vi "VarientToProperties.vi"(8 "error in (no error)":errorcluster, 11 "AcPwrPlugins.lvlib:NHRDCModel.lvclass":refnum<class "NHRDCPowerModel.lvclass">) -> (0 "error out":errorcluster, 1 "Measurements":T1, 2 "Device(s)Settings":T3 {"Modules"."Regulation Gain (1=100%)" min=0.0 max=1.0; "Modules"."OutputSettings"."Wait on Value" items=["Voltage Greater Than Or Equal To", "Voltage Less Than Or Equal To", "Current Greater Than Or Equal To", "Current Less Than Or Equal To", "Power Greater Than Or Equal To", "Power Less Than Or Equal To"]; "Modules"."operating state (Off)" items=["Off", "Stand By", "Charge", "Discharge", "Battery Emulation"]}, 3 "AcPwrPlugins.lvlib:NHRDCModel.lvclass":refnum<class "NHRDCPowerModel.lvclass">, 4 "Measurement Refresh Time (ms)":u32, 6 "Database Settings":T2)   [LabVIEW 2018, in "AcPwrPlugins.lvlib" / "NHRDCPowerModel.lvclass"]
uses:
  NHRDCPowerModel.lvclass
  NHRDCPowerClass/TypeDefs/Device(s)Settings.ctl
  NHRDCPowerClass/TypeDefs/Modules.ctl
  AcPwrShared/Database Settings.ctl
  NHRDCPowerClass/TypeDefs/Measurements.ctl
  F:/Projects/ICDAS/NistPluggableModules/AcPwr/AcPwrPlugins/AcPwrBaseClass/AcPwrBase.lvclass
  AcPwrBaseClass/AcPwrBase.lvclass/AcPwrBase.ctl
  AcPwrBaseClass/Accessors/Read BaseConfig.vi
  NHRDCPowerClass/NHRDCPower.lvclass
  AcPwrShared/AcPwrShared.lvlib
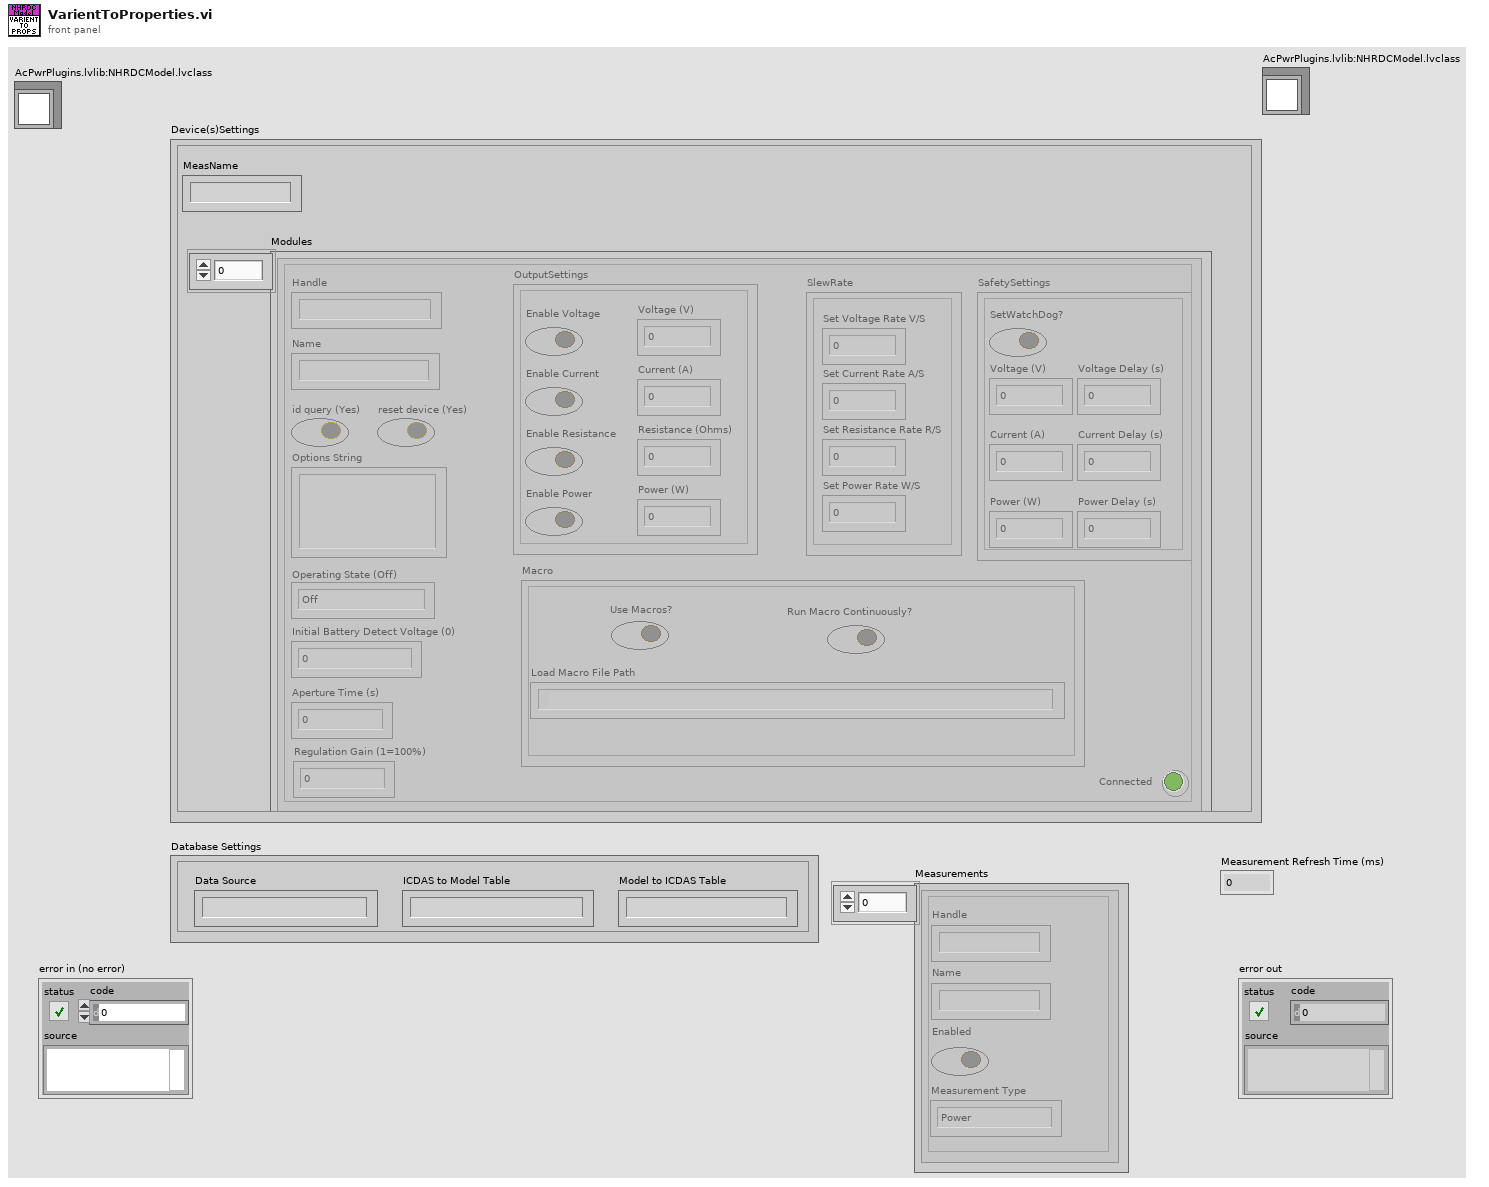
[diagram p1: front panel]
types:
  T1 = typedef "AcPwrPlugins.lvlib/NHRDCPower.lvclass/Measurements.ctl" = cluster{"Handle":string, "Name":string, "Enabled":bool, "Measurement Value":sgl, "Measurement Type":enum16{"Power", "Current", "Voltage"}}[]
  T2 = typedef "AcPwrShared.lvlib/Database Settings.ctl" = cluster{"Data Source":string, "ICDAS to Model Table":string, "Model to ICDAS Table":string}
  T3 = typedef "AcPwrPlugins.lvlib/NHRDCPower.lvclass/Device(s)Settings.ctl" = cluster{"MeasName":string, "Modules":T4}
  T4 = typedef "AcPwrPlugins.lvlib/NHRDCPower.lvclass/Modules.ctl" = cluster{"Handle":string, "Name":string, "id query (Yes)":bool, "reset device (Yes)":bool, "Connected":bool, "Initial Battery Detect Voltage (0)":dbl, "SafetySettings":cluster{"SetWatchDog?":bool, "Voltage (V)":dbl, "Current (A)":dbl, "Power (W)":dbl, "Voltage Delay (s)":dbl, "Current Delay (s)":dbl, "Power Delay (s)":dbl}, "Options String":string, "Aperture Time (s)":dbl, "operating state (Off)":i32, "OutputSettings":cluster{"Voltage (V)":dbl, "Current (A)":dbl, "Resistance (Ohms)":dbl, "Power (W)":dbl, "Enable Voltage":bool, "Enable Current":bool, "Enable Resistance":bool, "Enable Power":bool, "Macro After Step Delay  (s)":dbl, "Wait Value (V, A, W)":dbl, "Enable Wait":bool, "Wait on Value":i32}, "SlewRate":cluster{"Set Voltage Rate V/S":dbl, "Set Current Rate A/S":dbl, "Set Resistance Rate R/S":dbl, "Set Power Rate W/S":dbl}, "Macro":cluster{"Save Macro?":bool, "Load Macro From File?":bool, "Run Macro Continuously?":bool, "Use Macros?":bool, "Load Macro File Path":path, "Save Macro File Path":string}, "Regulation Gain (1=100%)":dbl, "UpdatingOntheFly":bool}[]
  T5 = typedef "AcPwrPlugins.lvlib/AcPwrBase.lvclass/BaseConfig.ctl" = cluster{"Frequency":dbl, "FrequencyRange":dbl[], "Phases":T6[], "Name":string, "PluginConfigVariant":variant, "PluginMeasVariant":variant}
  T6 = typedef "AcPwrPlugins.lvlib/AcPwrBase.lvclass/Phase.ctl" = cluster{"Name":string, "Enabled":bool, "VoltageLevel":dbl, "Handle":string, "VoltageRange":dbl[], "Connected":bool, "CurrentLimit":dbl, "Waveform":string}
  T7 = cluster{"Device(s)Settings":T3, "Database Settings":T2}
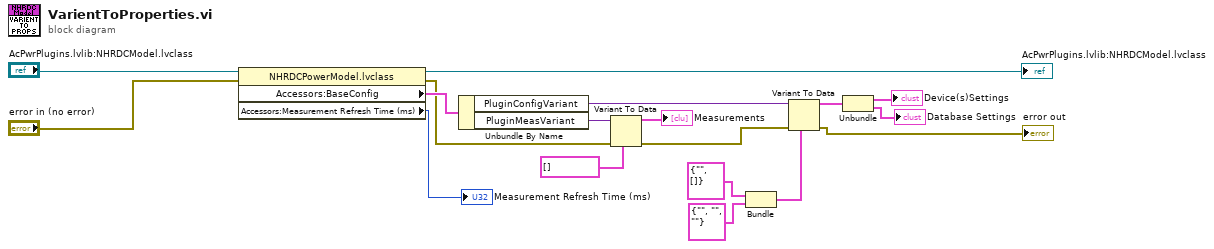
[diagram p0: block diagram]
diagram:
  n1 = property class="NHRDCPowerModel.lvclass"(reference="AcPwrPlugins.lvlib:NHRDCModel.lvclass", error in="error in (no error)") -> (reference out=→"AcPwrPlugins.lvlib:NHRDCModel.lvclass":refnum<class "NHRDCPowerModel.lvclass">, error out=w14:errorcluster, "Accessors:BaseConfig"=w16:T5, "Accessors:Measurement Refresh Time (ms)"=→"Measurement Refresh Time (ms)":u32)
  n2 = Unbundle By Name(w16) -> ("PluginConfigVariant"=w12:variant, "PluginMeasVariant"=w15:variant)
  n3 = Variant To Data(error in=w14, type=T1 [] ("Measurements"), Variant=w15) -> (data=→"Measurements":T1, error out=w11:errorcluster)
  n4 = Bundle("Device(s)Settings"=T3 {"MeasName"="", "Modules"=[]}, "Database Settings"=T2 {"Data Source"="", "ICDAS to Model Table"="", "Model to ICDAS Table"=""}) -> (w8:T7)  [unwired: 1 in]
  n5 = Variant To Data(error in=w11, type=w8, Variant=w12) -> (data=w7:T7, error out=→"error out":errorcluster)
  n6 = Unbundle(w7) -> ("Device(s)Settings"=→"Device(s)Settings":T3, "Database Settings"=→"Database Settings":T2)
